vi "svfa_Check Waveform Parameter Continuity (NxM) [Dual FFT].vi"(0 "stimulus signals X [EUx]":waveform(dbl)[](array[waveform]), 1 "restart averaging (F)":bool, 5 "response signals Y [EUy]":waveform(dbl)[](array[waveform]), 7 "checks for channel parameter change":T1, 9 "checks for multichannel parameters":T2, 11 "error in":errorcluster) -> (4 "dup stimulus signals X [EUx]":waveform(dbl)[](array[waveform]), 6 "dup response signals Y [EUy]":waveform(dbl)[](array[waveform]), 8 "waveform parameter changed":bool, 10 "multichannel parameter changed":bool, 15 "error out":errorcluster)   [LabVIEW 2017]
uses:
  <vilib>/addons/_NISVFA/_Shared subVIs/Common/svc_Check for Waveform Parameter Continuity (no state).vi
  <vilib>/addons/_NISVFA/_Shared subVIs/Common/svc_Get SV Channel Info.vi
  <vilib>/addons/_NISVFA/_Shared subVIs/Common/svc_Engineering Units to Unit Label.vi
  <vilib>/addons/_NISVFA/_Shared subVIs/Common/svc_Unit Label to Engineering Units.vi
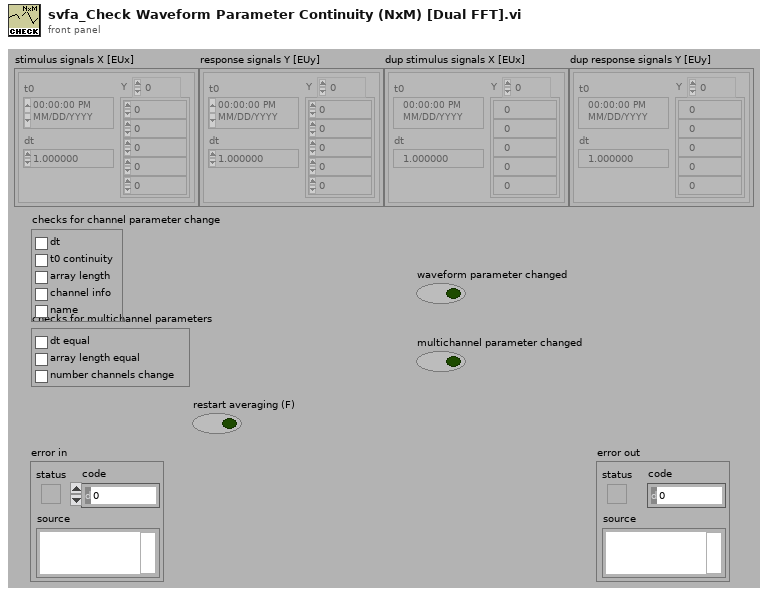
[diagram p1: front panel]
types:
  T1 = cluster{"dt":bool, "t0 continuity":bool, "array length":bool, "channel info":bool, "name":bool}
  T2 = cluster{"dt equal":bool, "array length equal":bool, "number channels change":bool}
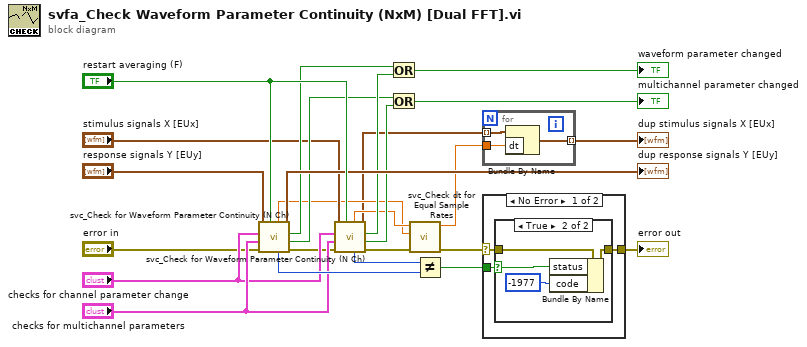
[diagram p0: block diagram]
diagram:
  n1 = call <vilib>:"svc_Check for Waveform Parameter Continuity (N Ch).vi"("restart averaging (F)"="restart averaging (F)", "error in (no error)"="error in", "checks for multichannel parameters"="checks for multichannel parameters", "checks for channel parameter change"="checks for channel parameter change", "scaled signal(s)"="response signals Y [EUy]") -> ("error out"=w21:errorcluster, "multichannel parameter changed"=w13:bool, "waveform parameter changed"=w16:bool, "dup scaled signal(s)"=→"dup response signals Y [EUy]":waveform(dbl)[], "array length"=w25:i32, "dt"=w6:dbl)  [unwired: 1 out]
  n2 = call <vilib>:"svc_Check for Waveform Parameter Continuity (N Ch).vi"("restart averaging (F)"="restart averaging (F)", "error in (no error)"=w21, "checks for multichannel parameters"="checks for multichannel parameters", "checks for channel parameter change"="checks for channel parameter change", "scaled signal(s)"="stimulus signals X [EUx]") -> ("error out"=w8:errorcluster, "multichannel parameter changed"=w14:bool, "waveform parameter changed"=w17:bool, "dup scaled signal(s)"=w3:waveform(dbl)[], "array length"=w24:i32, "dt"=w7:dbl)  [unwired: 1 out]
  n3 = Or(x=w16, y=w17) -> (x .or. y?=→"waveform parameter changed":bool)
  n4 = Or(x=w13, y=w14) -> (x .or. y?=→"multichannel parameter changed":bool)
  n5 = call <vilib>:"svc_Check dt for Equal Sample Rates.vi"("error in (no error)"=w8, "dt Y"=w6, "dt X"=w7) -> ("error out"=w9:errorcluster, "dt Y"=w1:dbl)  [unwired: 7 in]
  n6 = Not Equal?(x=w24, y=w25) -> (x != y?=w5:bool)
  n7 = for {
    tunnel: w3 -> [w28] mode=indexing
    tunnel: [w27] -> w2 mode=indexing
    tunnel: w1 -> [w26]
    n8 = Bundle By Name ("Build Waveform")(cluster=w28, "dt"=w26) -> (w27:waveform(dbl))
  }
  "dup stimulus signals X [EUx]" <- w2
  n9 = case shown="No Error" w9 {
    selector: w9 -> [w30 w37]
    tunnel: w5 -> [w31 _]
    tunnel: [w29 w37] -> w4
    frame No Error {
      n10 = case shown="True" w31 {
        selector: w31 -> [_ w34]
        tunnel: [w32 w36] -> w29
        tunnel: w30 -> [w32 w33]
        frame False {
        }
        frame True {
          n11 = Bundle By Name(cluster=w33, "status"=w34, "code"=-1977) -> (w36:errorcluster)
        }
      }
    }
    frame Error {
    }
  }
  "error out" <- w4
